vi "EventInPause_SM.vi"(0 "SM Private Data":refnum<class "Inspection Statemachine.lvclass">, 1 "LocalData_SM in":T1, 5 "Event Registration Refnum":refnum<event-registration>, 7 "CurrentState":string, 9 "Output Cluster":T2={"RackID"=0, "Trigger Light Camera Sequence"={"Light Sequence Trigger"="", "Status"="", "Mode"=""}, "Result Cluster"={"RackID"=0, "MeasurementValuesArray "=[], "ImagesArray"=[], "ResultPF"=FALSE, "ProductionCountDetails"={"TotalFail"=0, "TotalPass"=0, "TotalCount"=0}, "ReelCountDetails"={"ReelFail"=0, "ReelPass"=0, "ReelCount"=0}, "ControlPFArray"=[], "SpecificationPFArray"=[], "SpecificationFail"=FALSE, "ReelNumber"=0, "Status"=""}, "Analytics VI refnum"=refnum, "Statistical parameters "=[], "Sensor Name"="", "Camera Name"="", "PopupInput"={"Pop-up Type"=enum."Open Logo Display", "Title"="", "Message"="", "Button 1 Text"="", "Button 2 Text"="", "Show Close? T/F"=FALSE, "Title Blink? T/F"=FALSE, "Title Blink Colour"=0}, "PartInfo"={"PartName"="", "NumberOfRacks"=0, "TotalCount"=0, "ReelCount"=0, "OperatorName"="", "StampingMachineID"=0, "RackID"=0, "Reinitialize"=FALSE, "MeasurementNamesArray"=[], "MeasurementIDArray"=[], "SpecValuesArray"=[], "CameraNamesArray"=[]}, "StateMsgToMI"="", "InspectionStatusToMI"="", "StateMsgToRC"="", "StateMsgToUI"="", "StateMsgToDL"="", "StateMsgToAN"="", "StateMsgToSM"="", "EventData"={"EventName"="", "EventReason"=""}, "CameraOpticsDiagnosticsResult"={"LightCameraName"="", "DiagnosedImage"=refnum, "DustPercentage"=0.0, "Result"=TRUE}, "AllPartInfo"=[{"PartName"="", "NumberOfRacks"=0, "MeasurementIDsArray"=[], "MeasurementNamesArray"=[], "SpecValuesArray"=[]}], "SystemParameters"={"SystemName"="", "SystemID"="", "CustomerDetails"={"CustomerName"="", "CustomerId"="", "Location"="", "NumberOfShifts"=0.0, "ShiftDetails"=[]}, "InstallationDate"="", "NextServiceDate"="", "NumberOfRacks"=0, "TotalNumberOfCameras"=0, "SoftwareFeatures"={"HardwareEmulated"=FALSE, "PowerOnSelfTest"=FALSE, "DiagnosticsEnable"=FALSE, "AnalyticsEnable"=FALSE, "DefectTrackingEnable"=FALSE, "AutomaticGuideMovement"=FALSE, "DoorPokayokeEnable"=FALSE, "FailCountDisplayEnable"=FALSE, "FailCountReversalEnable"=FALSE, "DataLoggingEnable"=FALSE, "PauseOnReelCountFinish"=FALSE, "StopOnTotalCountFinish"=FALSE, "IoTEnable"=FALSE, "ReportEnable"=FALSE, "DebugLevel"=0.0, "PowerOnSelfTestFeatures"={"TimingUnit"=FALSE, "MachinePowerStatusCheck"=FALSE, "GuideMotor"=FALSE, "CameraOptics"=FALSE, "MasterSample"=FALSE}, "DiagnosticsFeatures"={"TimingUnit"=FALSE, "GuideMotor"=FALSE, "CameraOptics"=FALSE, "ReelerMotor"=FALSE, "HardwareButtons"=FALSE, "Sensors"=FALSE, "TowerLamp"=FALSE, "MasterSample"=FALSE}, "UserInterface"={"DynamicImageHandlingEnable"=FALSE, "DoorPokaYokeButtonVisible"=FALSE, "FailCountDisplayButtonVisible"=FALSE, "FailCountReversalButtonVisible"=FALSE}, "PopupOptions"={"ReasonForPause"=FALSE, "ReasonForFail"=FALSE, "ReasonForStop"=FALSE, "CpCpkOnReelFinish"=FALSE}, "DataloggingFeatures"={"EventData"=FALSE, "MeasurementData"=FALSE, "StatisticalData"=FALSE, "ReelData"=FALSE, "FailedMeasurementData"=FALSE, "FailedImages"=FALSE}, "IoT"={"SMSAlertEnable"=FALSE, "EmailAlertEnable"=FALSE}}}, "PartsConfigured"=[], "CameraSequenceList"=[], "SensorList"=[], "MasterSampleMessages"={"MasterSampleMessage"="", "PartMessage"=""}, "SensorDiagnosticsResult"={"Image Array"=[], "ImageCount"=0}, "IgnoredCountDetails"={"ReelCount"=0, "TotalCount"=0}, "MachineStatusToDL"="", "MasterSamplePartName"=""}, 11 "error in (no error)":errorcluster) -> (3 "LocalData_SM out":T1, 4 "NextState":string, 15 "error out":errorcluster)   [LabVIEW 2019, in "Inspection Statemachine.lvclass"]
uses:
  Inspection Statemachine.lvclass
  <vilib>/vision/Image Controls.llb/IMAQ Image.ctl
  Controls/Result Cluster_SM.ctl
  Common/Controls/Camera Optics Diagnostics Result.ctl
  Common/Controls/Pop-up Input.ctl
  Controls/Output Cluster_SM.ctl
  Common/Controls/AllPartInfo.ctl
  Controls/LocalData_SM.ctl
  Common/Controls/Diagnostics Result.ctl
  <vilib>/ActorFramework/Message Enqueuer/Message Enqueuer.lvclass
  Common/Controls/Acknowledgement.ctl
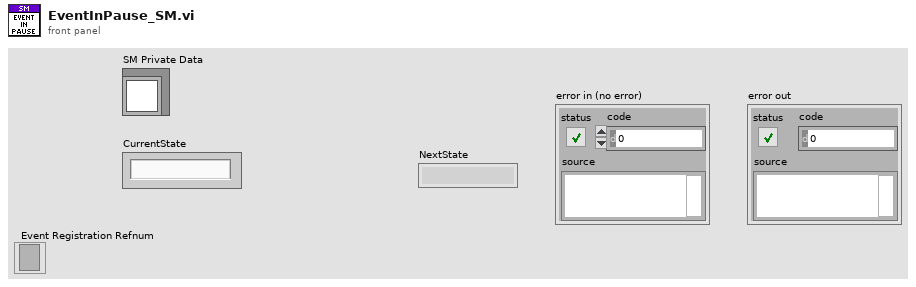
[diagram p1: front panel]
types:
  T1 = typedef "Inspection Statemachine.lvclass/LocalData_SM.ctl" = cluster{"Timeout":i32, "Core":cluster{"Current VI Reference":refnum<vi>, "Close Panel on Exit?":bool}, "Ack":u8, " CurrentState":string, "DirectExit":bool, "SoftwareExit":bool, "SensorDiagnosticsStatus":bool, "OutputCluster":T2, "SelComplete":bool, "ResultToMI":bool, "Exit":bool, "NumberOfActorsLaunched":i32, "BatchStart":bool, "LoadingBarActive":bool, "UpdateInPause":bool, " EventReason":string, "PopUpCategory":string, "PopUpActive":bool, "MasterSampleState":string, "CameraOpticsDiagnosticsStatus":bool, "CameraIndex":i32, "SensorIndex":i32}
  T2 = typedef "Inspection Statemachine.lvclass/Output Cluster_SM.ctl" = cluster{"RackID":u8, "Trigger Light Camera Sequence":cluster{"Light Sequence Trigger":string, "Status":string, "Mode":string}, "Result Cluster":T3, "Analytics VI refnum":refnum<vi>, "Statistical parameters ":string[][], "Sensor Name":string, "Camera Name":string, "PopupInput":T5, "PartInfo":cluster{"PartName":string, "NumberOfRacks":u8, "TotalCount":u64, "ReelCount":u64, "OperatorName":string, "StampingMachineID":u32, "RackID":u8, "Reinitialize":bool, "MeasurementNamesArray":string[], "MeasurementIDArray":u16[], "SpecValuesArray":cluster{"LCL":dbl, "UCL":dbl, "LSL":dbl, "USL":dbl, "Nominal Value":dbl}[], "CameraNamesArray":string[]}, "StateMsgToMI":string, "InspectionStatusToMI":string, "StateMsgToRC":string, "StateMsgToUI":string, "StateMsgToDL":string, "StateMsgToAN":string, "StateMsgToSM":string, "EventData":cluster{"EventName":string, "EventReason":string}, "CameraOpticsDiagnosticsResult":T6, "AllPartInfo":T7, "SystemParameters":cluster{"SystemName":string, "SystemID":string, "CustomerDetails":cluster{"CustomerName":string, "CustomerId":string, "Location":string, "NumberOfShifts":dbl, "ShiftDetails":cluster{"Name":string, "Timing":string}[]}, "InstallationDate":string, "NextServiceDate":string, "NumberOfRacks":u8, "TotalNumberOfCameras":u8, "SoftwareFeatures":cluster{"HardwareEmulated":bool, "PowerOnSelfTest":bool, "DiagnosticsEnable":bool, "AnalyticsEnable":bool, "DefectTrackingEnable":bool, "AutomaticGuideMovement":bool, "DoorPokayokeEnable":bool, "FailCountDisplayEnable":bool, "FailCountReversalEnable":bool, "DataLoggingEnable":bool, "PauseOnReelCountFinish":bool, "StopOnTotalCountFinish":bool, "IoTEnable":bool, "ReportEnable":bool, "DebugLevel":dbl, "PowerOnSelfTestFeatures":cluster{"TimingUnit":bool, "MachinePowerStatusCheck":bool, "GuideMotor":bool, "CameraOptics":bool, "MasterSample":bool}, "DiagnosticsFeatures":cluster{"TimingUnit":bool, "GuideMotor":bool, "CameraOptics":bool, "ReelerMotor":bool, "HardwareButtons":bool, "Sensors":bool, "TowerLamp":bool, "MasterSample":bool}, "UserInterface":cluster{"DynamicImageHandlingEnable":bool, "DoorPokaYokeButtonVisible":bool, "FailCountDisplayButtonVisible":bool, "FailCountReversalButtonVisible":bool}, "PopupOptions":cluster{"ReasonForPause":bool, "ReasonForFail":bool, "ReasonForStop":bool, "CpCpkOnReelFinish":bool}, "DataloggingFeatures":cluster{"EventData":bool, "MeasurementData":bool, "StatisticalData":bool, "ReelData":bool, "FailedMeasurementData":bool, "FailedImages":bool}, "IoT":cluster{"SMSAlertEnable":bool, "EmailAlertEnable":bool}}}, "PartsConfigured":cluster{"Name":string, "NumberOfRack":u8}[], "CameraSequenceList":cluster{"Name":string, "RackID":u8}[], "SensorList":cluster{"Name":string, "RackID":u8}[], "MasterSampleMessages":cluster{"MasterSampleMessage":string, "PartMessage":string}, "SensorDiagnosticsResult":cluster{"Image Array":T4[], "ImageCount":u64}, "IgnoredCountDetails":cluster{"ReelCount":u64, "TotalCount":u64}, "MachineStatusToDL":string, "MasterSamplePartName":string}
  T3 = typedef "Inspection Statemachine.lvclass/Result Cluster_SM.ctl" = cluster{"RackID":u8, "MeasurementValuesArray ":dbl[], "ImagesArray":T4[], "ResultPF":bool, "ProductionCountDetails":cluster{"TotalFail":u64, "TotalPass":u64, "TotalCount":u64}, "ReelCountDetails":cluster{"ReelFail":u64, "ReelPass":u64, "ReelCount":u64}, "ControlPFArray":bool[], "SpecificationPFArray":bool[], "SpecificationFail":bool, "ReelNumber":u64, "Status":string}
  T4 = typedef "IMAQ Image.ctl" = refnum<image>
  T5 = typedef "Pop-up Input.ctl" = cluster{"Pop-up Type":enum16{"Open Logo Display", "Close Logo Display", "Open Loading Bar", "Close Loading Bar", "Open Alert Display", "Close Alert Display", "One button dialog box", "Two button dialog box", "User Authentication"}, "Title":string, "Message":string, "Button 1 Text":string, "Button 2 Text":string, "Show Close? T/F":bool, "Title Blink? T/F":bool, "Title Blink Colour":u32}
  T6 = typedef "Camera Optics Diagnostics Result.ctl" = cluster{"LightCameraName":string, "DiagnosedImage":T4, "DustPercentage":dbl, "Result":bool}
  T7 = typedef "AllPartInfo.ctl" = cluster{"PartName":string, "NumberOfRacks":u8, "MeasurementIDsArray":u16[], "MeasurementNamesArray":string[], "SpecValuesArray":cluster{"LCL":dbl, "UCL":dbl, "LSL":dbl, "USL":dbl, "NominalValue":dbl}[]}[]
  T8 = enum16{"Open Logo Display", "Close Logo Display", "Open Loading Bar", "Close Loading Bar", "Open Alert Display", "Close Alert Display", "One button dialog box", "Two button dialog box", "User Authentication"}
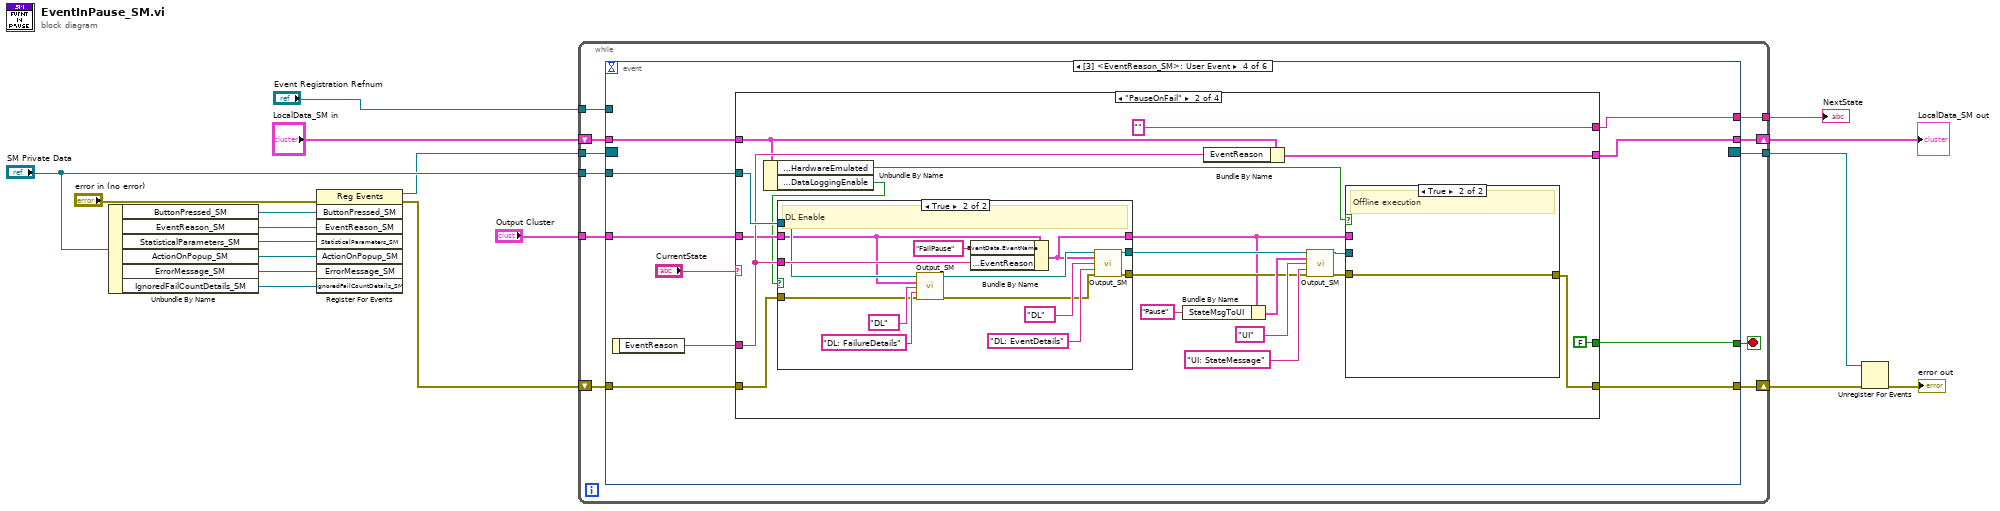
[diagram p0: block diagram]
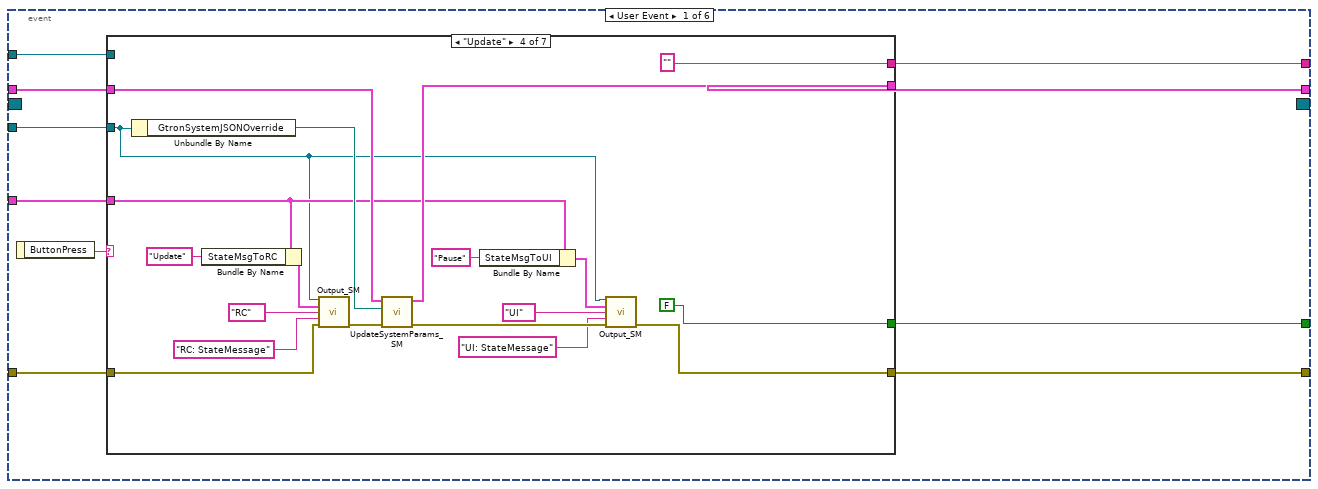
[diagram p2: hidden frame]
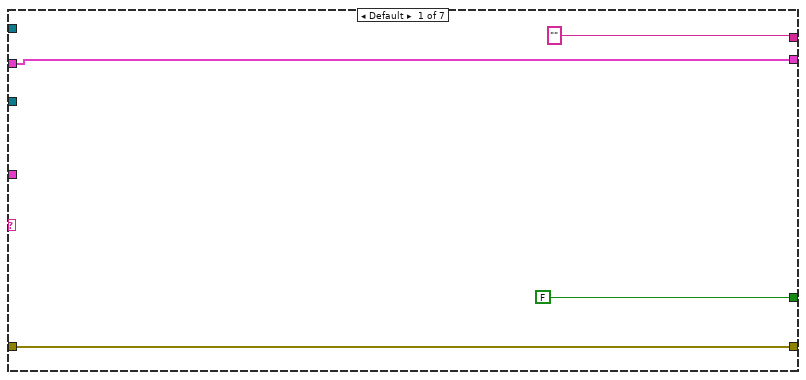
[diagram p3: hidden frame]
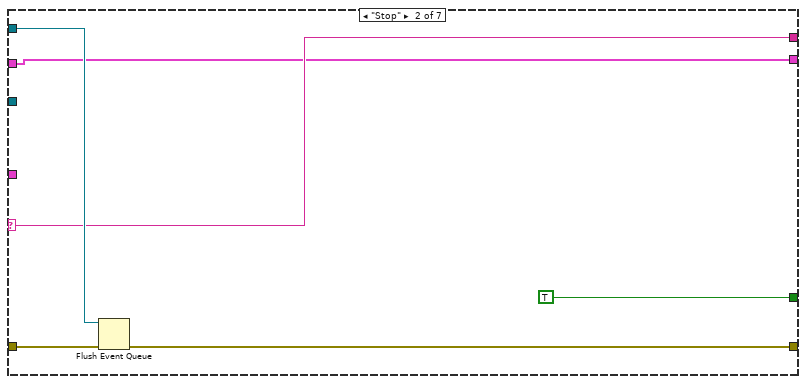
[diagram p4: hidden frame]
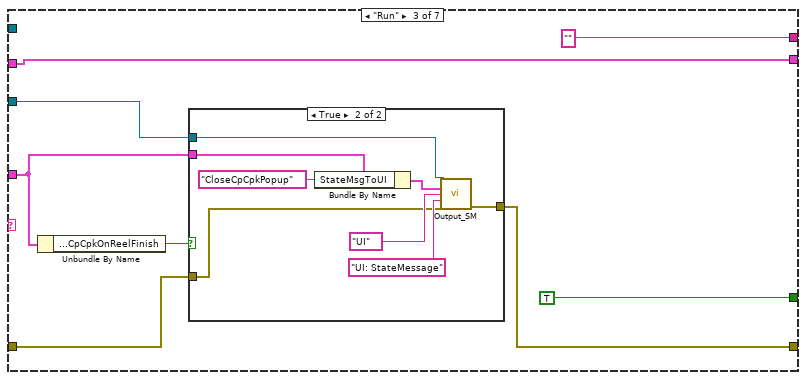
[diagram p5: hidden frame]
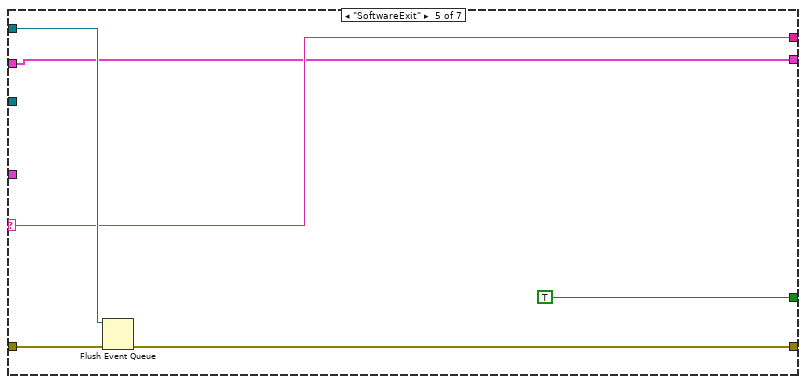
[diagram p7: hidden frame]
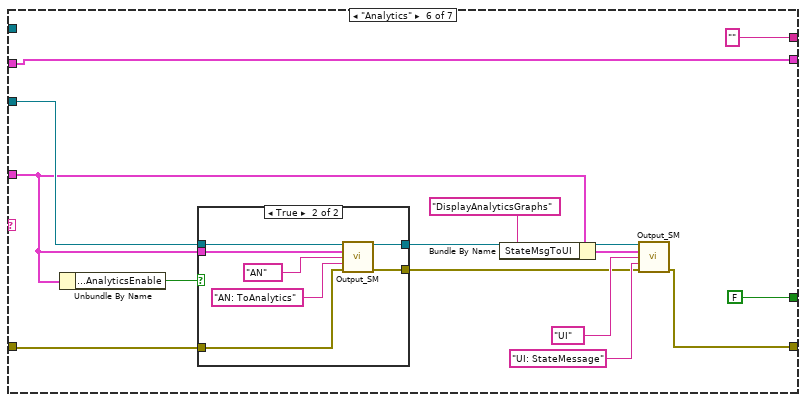
[diagram p8: hidden frame]
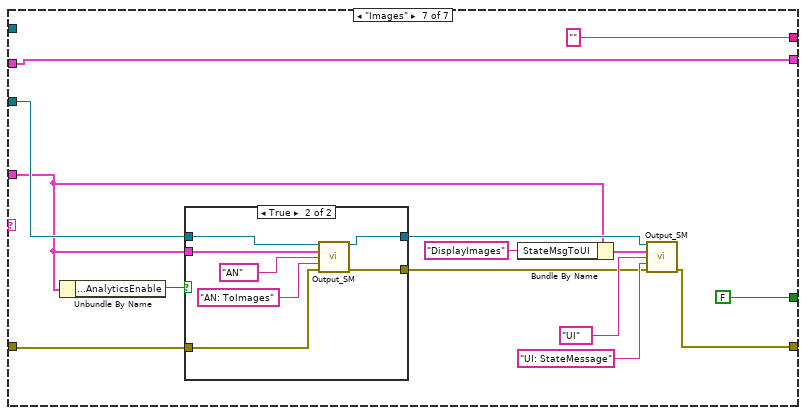
[diagram p10: hidden frame]
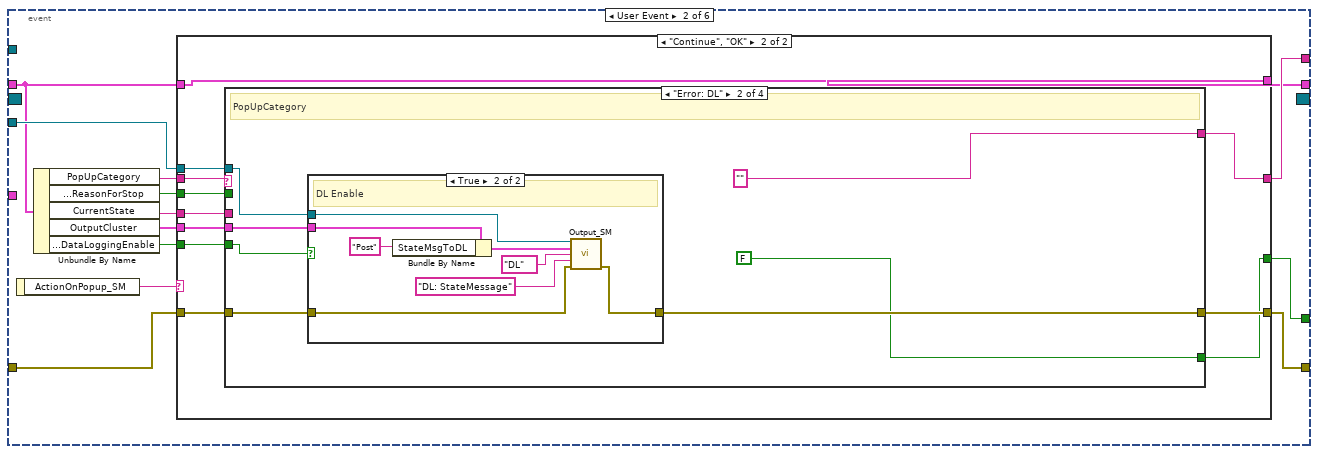
[diagram p12: hidden frame]
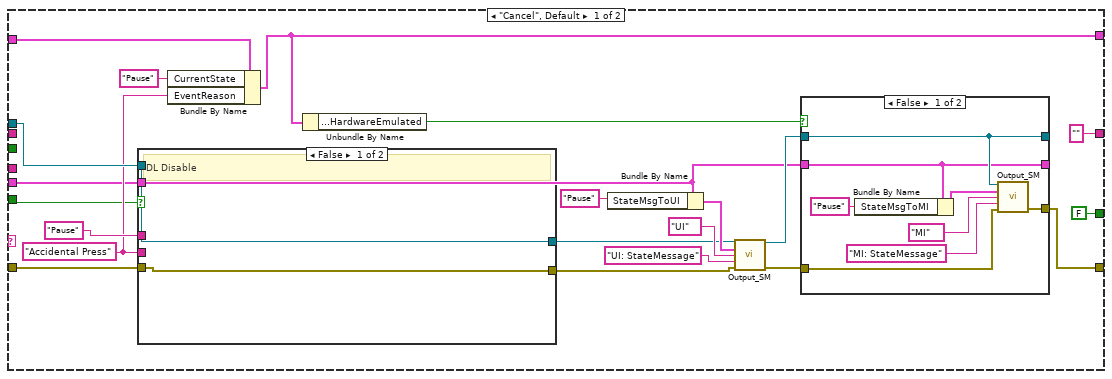
[diagram p13: hidden frame]
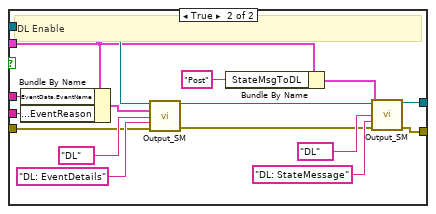
[diagram p14: hidden frame]
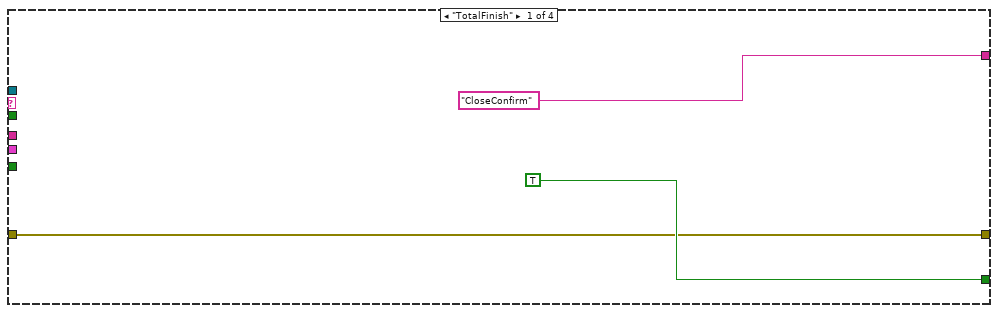
[diagram p16: hidden frame]
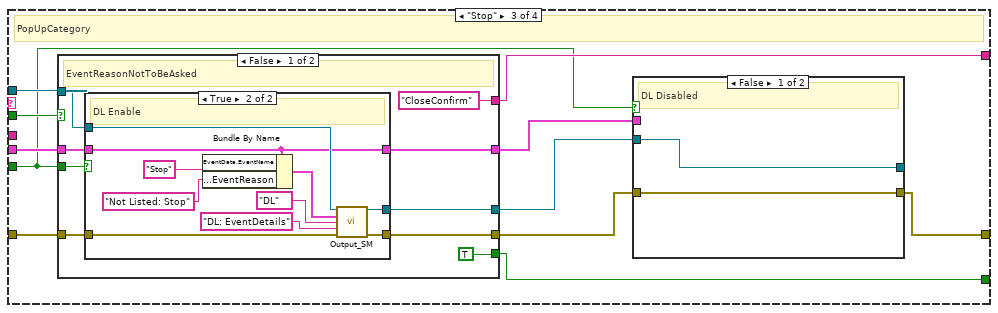
[diagram p18: hidden frame]
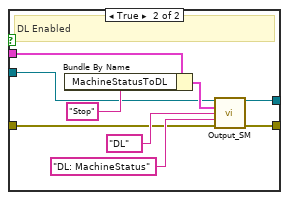
[diagram p19: hidden frame]
diagram:
  n1 = Unbundle By Name("SM Private Data") -> ("ButtonPressed_SM"=w14:refnum<user-event>, "EventReason_SM"=w13:refnum<user-event>, "StatisticalParameters_SM"=w12:refnum<user-event>, "ActionOnPopup_SM"=w4:refnum<user-event>, "ErrorMessage_SM"=w2:refnum<user-event>, "IgnoredFailCountDetails_SM"=w1:refnum<user-event>)
  n2 = register-events(error in="error in (no error)", w14, w13, w12, w4, w2, w1) -> (reference out=w10:refnum<event-registration>, error out=w8:errorcluster)  [unwired: 1 in]
  n3 = while {
    tunnel: w10 -> [w29]
    tunnel: [w28] -> w17
    tunnel: [w23] -> w18
    tunnel: "Event Registration Refnum" -> [w24]
    tunnel: "SM Private Data" -> [w22]
    tunnel: "Output Cluster" -> [w21]
    shift-right: [w25] -> w16
    shift-left: w8 -> [w26]
    shift-right: [w19] -> w5
    shift-left: "LocalData_SM in" -> [w20]
    stop <- w27 stop-if-true
    n4 = event shown="[3] <EventReason_SM>: User Event" {
      selector: w29 -> [_ _ _ _ _ _]
      dyn-events: [_ _ _ _ _ _] -> w28
      timeout: _ -> [_ _ _ _ _ _]
      tunnel: [w35 w142 FALSE w323 _ FALSE] -> w27
      tunnel: w26 -> [w39 w149 w298 w327 w439 w488]
      tunnel: [w38 w150 w297 w324 w443 w487] -> w25
      tunnel: w24 -> [w36 _ _ _ _ _]
      tunnel: [w34 w143 "" w322 "" ""] -> w23
      tunnel: w22 -> [w33 w144 w296 w326 w440 w485]
      tunnel: w21 -> [w32 _ w299 w325 w448 _]
      tunnel: w20 -> [w31 w141 w292 w321 w452 w484]
      tunnel: [w30 w140 w291 w320 w452 w484] -> w19
      event User Event {
        n5 = event-data() -> ("ButtonPress"=w37:string)  [unwired: 1 in]
        n6 = case shown="\"Update\"" w37 {
          selector: w37 -> [_ w46 _ _ w87 _ _]
          tunnel: w39 -> [w43 w49 w52 w84 w90 w101 w124]
          tunnel: [w43 w45 w51 w73 w89 w100 w123] -> w38
          tunnel: w36 -> [_ w48 _ _ w88 _ _]
          tunnel: [FALSE TRUE TRUE FALSE TRUE FALSE FALSE] -> w35
          tunnel: ["" w46 "" "" w87 "" ""] -> w34
          tunnel: w33 -> [_ _ w53 w67 _ w95 w118]
          tunnel: w32 -> [_ _ w50 w71 _ w93 w116]
          tunnel: w31 -> [w40 w44 w55 w77 w86 w96 w119]
          tunnel: [w40 w44 w55 w76 w86 w96 w119] -> w30
          frame Default {
          }
          frame "Stop" {
            n7 = Flush Event Queue(0:w48, 3:w49) -> (11:w45:errorcluster)  [unwired: 4 in, 2 out]
          }
          frame "Run" {
            n8 = Unbundle By Name(w50) -> ("SystemParameters.SoftwareFeatures.PopupOptions.CpCpkOnReelFinish"=w54:bool)
            n9 = case shown="True" w54 {
              tunnel: w53 -> [_ w64]
              tunnel: w52 -> [w58 w63]
              tunnel: [w58 w62] -> w51
              tunnel: w50 -> [_ w61]
              frame False {
              }
              frame True {
                n10 = Bundle By Name(cluster=w61, "StateMsgToUI"="CloseCpCpkPopup" ("StateMsgToSM")) -> (w60:T2)
                n11 = call "Output_SM.vi"("SM Private Data in"=w64, "Output Cluster"=w60, "Receiver Name"="UI", "State"="UI: StateMessage", "error in (no error)"=w63) -> ("error out"=w62:errorcluster)  [unwired: 9 in, 1 out]
              }
            }
          }
          frame "Update" {
            n12 = Unbundle By Name(w67) -> ("GtronSystemJSONOverride"=w75:path)
            n13 = Bundle By Name(cluster=w71, "StateMsgToRC"="Update") -> (w81:T2)
            n14 = call "Output_SM.vi"("SM Private Data in"=w67, "Output Cluster"=w81, "Receiver Name"="RC", "State"="RC: StateMessage", "error in (no error)"=w84) -> ("error out"=w78:errorcluster)  [unwired: 9 in, 1 out]
            n15 = call "UpdateSystemParams_SM.vi"("error in (no error)"=w78, "Override File Path"=w75, "Cluster In"=w77) -> ("error out"=w74:errorcluster, "Cluster Out"=w76:T1)  [unwired: 7 in]
            n16 = Bundle By Name(cluster=w71, "StateMsgToUI"="Pause") -> (w70:T2)
            n17 = call "Output_SM.vi"("SM Private Data in"=w67, "Output Cluster"=w70, "Receiver Name"="UI", "State"="UI: StateMessage", "error in (no error)"=w74) -> ("error out"=w73:errorcluster)  [unwired: 9 in, 1 out]
          }
          frame "SoftwareExit" {
            n18 = Flush Event Queue(0:w88, 3:w90) -> (11:w89:errorcluster)  [unwired: 4 in, 2 out]
          }
          frame "Analytics" {
            n19 = Unbundle By Name(w93) -> ("SystemParameters.SoftwareFeatures.AnalyticsEnable"=w92:bool)
            n20 = case shown="True" w92 {
              tunnel: [w106 w114] -> w103
              tunnel: w101 -> [w106 w111]
              tunnel: w95 -> [w107 w110]
              tunnel: w93 -> [_ w109]
              tunnel: [w107 w108] -> w94
              frame False {
              }
              frame True {
                n21 = call "Output_SM.vi"("SM Private Data in"=w110, "Output Cluster"=w109, "Receiver Name"="AN", "State"="AN: ToAnalytics", "error in (no error)"=w111) -> ("SM Private Data out"=w108:refnum<class "Inspection Statemachine.lvclass">, "error out"=w114:errorcluster)  [unwired: 9 in]
              }
            }
            n22 = Bundle By Name(cluster=w93, "StateMsgToUI"="DisplayAnalyticsGraphs") -> (w97:T2)
            n23 = call "Output_SM.vi"("SM Private Data in"=w94, "Output Cluster"=w97, "Receiver Name"="UI", "State"="UI: StateMessage", "error in (no error)"=w103) -> ("error out"=w100:errorcluster)  [unwired: 9 in, 1 out]
          }
          frame "Images" {
            n24 = Unbundle By Name(w116) -> ("SystemParameters.SoftwareFeatures.AnalyticsEnable"=w115:bool)
            n25 = case shown="True" w115 {
              tunnel: [w129 w137] -> w126
              tunnel: w124 -> [w129 w134]
              tunnel: w116 -> [_ w133]
              tunnel: w118 -> [w130 w132]
              tunnel: [w130 w131] -> w117
              frame False {
              }
              frame True {
                n26 = call "Output_SM.vi"("SM Private Data in"=w132, "Output Cluster"=w133, "Receiver Name"="AN", "State"="AN: ToImages", "error in (no error)"=w134) -> ("SM Private Data out"=w131:refnum<class "Inspection Statemachine.lvclass">, "error out"=w137:errorcluster)  [unwired: 9 in]
              }
            }
            n27 = Bundle By Name(cluster=w116, "StateMsgToUI"="DisplayImages") -> (w120:T2)
            n28 = call "Output_SM.vi"("SM Private Data in"=w117, "Output Cluster"=w120, "Receiver Name"="UI", "State"="UI: StateMessage", "error in (no error)"=w126) -> ("error out"=w123:errorcluster)  [unwired: 9 in, 1 out]
          }
        }
      }
      event User Event {
        n29 = event-data() -> ("ActionOnPopup_SM"=w148:string)  [unwired: 1 in]
        n30 = Unbundle By Name(w141) -> ("PopUpCategory"=w139:string, "OutputCluster.SystemParameters.SoftwareFeatures.PopupOptions.ReasonForStop"=w145:bool, "CurrentState"=w146:string, "OutputCluster"=w147:T2, "OutputCluster.SystemParameters.SoftwareFeatures.DataLoggingEnable"=w138:bool)
        n31 = case shown="\"Continue\", \"OK\"" w148 {
          tunnel: ["" w211] -> w143
          tunnel: w146 -> [_ w210]
          tunnel: w147 -> [w153 w209]
          tunnel: w144 -> [w161 w208]
          tunnel: w149 -> [w162 w207]
          tunnel: [w155 w206] -> w150
          tunnel: w145 -> [_ w205]
          tunnel: [FALSE w204] -> w142
          tunnel: w141 -> [w165 w203]
          tunnel: [w157 w203] -> w140
          tunnel: w139 -> [_ w202]
          tunnel: w138 -> [w151 w201]
          frame "Cancel", Default {
            w160 = "Accidental Press" ("EventReason")
            n32 = case shown="False" w151 {
              tunnel: "Pause" ("DataLogger.EventDetails.EventName") -> [_ w187]
              tunnel: w162 -> [w172 w185]
              tunnel: w161 -> [w173 w184]
              tunnel: w160 -> [_ w183]
              tunnel: [w173 w177] -> w154
              tunnel: w153 -> [_ w175]
              tunnel: [w172 w174] -> w152
              frame False {
                # "DL Disable"
              }
              frame True {
                # "DL Enable"
                n33 = Bundle By Name(cluster=w175, "EventData.EventName"=w187, "EventData.EventReason"=w183) -> (w188:T2)
                n34 = call "Output_SM.vi"("SM Private Data in"=w184, "Output Cluster"=w188, "Receiver Name"="DL", "State"="DL: EventDetails", "error in (no error)"=w185) -> ("SM Private Data out"=w178:refnum<class "Inspection Statemachine.lvclass">, "error out"=w176:errorcluster)  [unwired: 9 in]
                n35 = Bundle By Name(cluster=w175, "StateMsgToDL"="Post") -> (w180:T2)
                n36 = call "Output_SM.vi"("SM Private Data in"=w178, "Output Cluster"=w180, "Receiver Name"="DL", "State"="DL: StateMessage", "error in (no error)"=w176) -> ("SM Private Data out"=w177:refnum<class "Inspection Statemachine.lvclass">, "error out"=w174:errorcluster)  [unwired: 9 in]
              }
            }
            n37 = Bundle By Name(cluster=w165, "CurrentState"="Pause", "EventReason"=w160) -> (w157:T1)
            n38 = Unbundle By Name(w157) -> ("OutputCluster.SystemParameters.SoftwareFeatures.HardwareEmulated"=w156:bool)
            n39 = Bundle By Name(cluster=w153, "StateMsgToUI"="Pause" ("StateMsgToRC")) -> (w167:T2)
            n40 = call "Output_SM.vi"("SM Private Data in"=w154, "Output Cluster"=w167, "Receiver Name"="UI", "State"="UI: StateMessage", "error in (no error)"=w152) -> ("SM Private Data out"=w158:refnum<class "Inspection Statemachine.lvclass">, "error out"=w159:errorcluster)  [unwired: 9 in]
            n41 = case shown="False" w156 {
              tunnel: w153 -> [w190 w198]
              tunnel: w158 -> [w191 w199]
              tunnel: w159 -> [w193 w200]
              tunnel: [w192 w200] -> w155
              tunnel: [w191 w199] -> _
              tunnel: [w190 w198] -> _
              frame False {
                n42 = Bundle By Name(cluster=w190, "StateMsgToMI"="Pause") -> (w195:T2)
                n43 = call "Output_SM.vi"("SM Private Data in"=w191, "Output Cluster"=w195, "Receiver Name"="MI", "State"="MI: StateMessage", "error in (no error)"=w193) -> ("error out"=w192:errorcluster)  [unwired: 9 in, 1 out]
              }
              frame True {
              }
            }
          }
          frame "Continue", "OK" {
            n44 = case shown="\"Error: DL\"" w202 {
              tunnel: ["CloseConfirm" "" w241 ""] -> w211
              tunnel: w210 -> [_ _ _ _]
              tunnel: w209 -> [_ w220 w240 _]
              tunnel: w208 -> [_ w219 w239 _]
              tunnel: w207 -> [w212 w218 w238 w288]
              tunnel: [w212 w217 w235 w288] -> w206
              tunnel: w205 -> [_ _ w237 _]
              tunnel: [TRUE FALSE w236 FALSE] -> w204
              tunnel: w201 -> [_ w215 w231 _]
              frame "TotalFinish" {
              }
              frame "Error: DL" {
                # "PopUpCategory"
                n45 = case shown="True" w215 {
                  tunnel: w220 -> [_ w230]
                  tunnel: w219 -> [_ w229]
                  tunnel: w218 -> [w222 w228]
                  tunnel: [w222 w227] -> w217
                  frame False {
                    # "DL DIsable"
                  }
                  frame True {
                    # "DL Enable"
                    n46 = Bundle By Name(cluster=w230, "StateMsgToDL"="Post") -> (w225:T2)
                    n47 = call "Output_SM.vi"("SM Private Data in"=w229, "Output Cluster"=w225, "Receiver Name"="DL", "State"="DL: StateMessage", "error in (no error)"=w228) -> ("error out"=w227:errorcluster)  [unwired: 9 in, 1 out]
                  }
                }
              }
              frame "Stop" {
                # "PopUpCategory"
                n48 = case shown="False" w237 {
                  tunnel: w238 -> [w259 w277]
                  tunnel: [w260 w284] -> w234
                  tunnel: w240 -> [w258 w275]
                  tunnel: w239 -> [w261 w278]
                  tunnel: ["CloseConfirm" ""] -> w241
                  tunnel: [TRUE FALSE] -> w236
                  tunnel: w231 -> [w255 _]
                  tunnel: [w254 w276] -> w233
                  tunnel: [w253 w275] -> w232
                  frame False {
                    # "EventReasonNotToBeAsked"
                    n49 = case shown="True" w255 {
                      tunnel: w261 -> [w262 w270]
                      tunnel: [w264 w269] -> w260
                      tunnel: w259 -> [w264 w268]
                      tunnel: w258 -> [w263 w265]
                      tunnel: [w262 w266] -> w254
                      tunnel: [w263 w265] -> w253
                      frame False {
                        # "DL Disable"
                      }
                      frame True {
                        # "DL Enable"
                        n50 = Bundle By Name(cluster=w265, "EventData.EventName"="Stop" ("DataLogger.EventDetails.EventName"), "EventData.EventReason"="Not Listed: Stop") -> (w272:T2)
                        n51 = call "Output_SM.vi"("SM Private Data in"=w270, "Output Cluster"=w272, "Receiver Name"="DL", "State"="DL: EventDetails", "error in (no error)"=w268) -> ("SM Private Data out"=w266:refnum<class "Inspection Statemachine.lvclass">, "error out"=w269:errorcluster)  [unwired: 9 in]
                      }
                    }
                  }
                  frame True {
                    # "EventReasonToBeAsked"
                    n52 = Bundle By Name(cluster=w275, "StateMsgToUI"="Stop") -> (w282:T2)
                    n53 = call "Output_SM.vi"("SM Private Data in"=w278, "Output Cluster"=w282, "Receiver Name"="UI", "State"="UI: AskEventReason", "error in (no error)"=w277) -> ("SM Private Data out"=w276:refnum<class "Inspection Statemachine.lvclass">, "error out"=w284:errorcluster)  [unwired: 9 in]
                  }
                }
                n54 = case shown="False" w231 {
                  tunnel: w234 -> [w242 w248]
                  tunnel: w233 -> [w243 w247]
                  tunnel: w232 -> [_ w246]
                  tunnel: [w242 w245] -> w235
                  tunnel: [w243 w244] -> _
                  frame False {
                    # "DL Disabled"
                  }
                  frame True {
                    # "DL Enabled"
                    n55 = Bundle By Name(cluster=w246, "MachineStatusToDL"="Stop" ("StateMsgToDL")) -> (w251:T2)
                    n56 = call "Output_SM.vi"("SM Private Data in"=w247, "Output Cluster"=w251, "Receiver Name"="DL", "State"="DL: MachineStatus", "error in (no error)"=w248) -> ("SM Private Data out"=w244:refnum<class "Inspection Statemachine.lvclass">, "error out"=w245:errorcluster)  [unwired: 9 in]
                  }
                }
              }
              frame Default {
              }
            }
          }
        }
      }
      event User Event {
        n57 = event-data() -> ("ErrorMessage"=w294:string)  [unwired: 1 in]
        n58 = Match Pattern(string=w294, regular expression="_") -> (before substring=w293:string)  [unwired: 1 in, 3 out]
        n59 = case shown="\"DataLogger\"" w293 {
          tunnel: w299 -> [_ w304]
          tunnel: w298 -> [w300 w311]
          tunnel: [w300 w310] -> w297
          tunnel: w296 -> [_ w309]
          tunnel: w292 -> [w301 w306]
          tunnel: [w301 w305] -> w291
          frame Default {
          }
          frame "DataLogger" {
            n60 = Bundle By Name(cluster=w306, "DirectExit"=FALSE ("Direct Exit"), "SoftwareExit"=FALSE ("Software Exit?"), "PopUpCategory"="Error: DL", "PopUpActive"=TRUE) -> (w305:T1)
            n61 = Bundle By Name(cluster=w304, "PopupInput.Title"="ALERT!" ("title"), "PopupInput.Message"="File Open!\nUnable To Write.Please Close Data File." ("string"), "PopupInput.Title Blink? T/F"=TRUE ("title blink?"), "PopupInput.Button 1 Text"="OK", "PopupInput.Pop-up Type"=T8."One button dialog box") -> (w314:T2)
            n62 = call "Output_SM.vi"("SM Private Data in"=w309, "Output Cluster"=w314, "Receiver Name"="UI", "State"="UI: DisplayPopup", "error in (no error)"=w311) -> ("error out"=w310:errorcluster)  [unwired: 9 in, 1 out]
          }
        }
      }
      event User Event {
        n63 = event-data() -> ("EventReason"=w328:string)  [unwired: 1 in]
        n64 = case shown="\"PauseOnFail\"" "CurrentState" {
          tunnel: w328 -> [w333 w359 w402 _]
          tunnel: w327 -> [w334 w368 w413 w438]
          tunnel: w326 -> [w335 w367 w412 _]
          tunnel: w325 -> [w331 w352 w397 _]
          tunnel: [w338 w354 w400 w438] -> w324
          tunnel: [TRUE FALSE FALSE FALSE] -> w323
          tunnel: ["CloseConfirm" "" "" ""] -> w322
          tunnel: w321 -> [w332 w358 w403 w435]
          tunnel: [w332 w360 w399 w435] -> w320
          frame "Stop" {
            n65 = Unbundle By Name(w331) -> ("SystemParameters.SoftwareFeatures.DataLoggingEnable"=w330:bool)
            n66 = case shown="False" w330 {
              tunnel: [w339 w344] -> w338
              tunnel: w335 -> [_ w343]
              tunnel: w331 -> [_ w342]
              tunnel: w334 -> [w339 w341]
              tunnel: w333 -> [_ w340]
              frame False {
                # "DL Disable"
              }
              frame True {
                # "DL Enable"
                n67 = Bundle By Name(cluster=w342, "EventData.EventName"="Stop" ("DataLogger.EventDetails.EventName"), "EventData.EventReason"=w340) -> (w346:T2)
                n68 = call "Output_SM.vi"("SM Private Data in"=w343, "Output Cluster"=w346, "Receiver Name"="DL", "State"="DL: EventDetails", "error in (no error)"=w341) -> ("error out"=w344:errorcluster)  [unwired: 9 in, 1 out]
              }
            }
          }
          frame "PauseOnFail" {
            n69 = Unbundle By Name(w358) -> ("OutputCluster.SystemParameters.SoftwareFeatures.HardwareEmulated"=w357:bool, "OutputCluster.SystemParameters.SoftwareFeatures.DataLoggingEnable"=w350:bool)
            n70 = case shown="True" w350 {
              tunnel: w368 -> [w371 w377]
              tunnel: w367 -> [w369 w375]
              tunnel: w359 -> [_ w382]
              tunnel: [w369 w380] -> w353
              tunnel: w352 -> [w370 w373]
              tunnel: [w371 w381] -> w351
              tunnel: [w370 w372] -> w349
              frame False {
                # "DL Disable"
              }
              frame True {
                # "DL Enable"
                n71 = call "Output_SM.vi"("SM Private Data in"=w375, "Output Cluster"=w373, "Receiver Name"="DL", "State"="DL: FailureDetails", "error in (no error)"=w377) -> ("SM Private Data out"=w374:refnum<class "Inspection Statemachine.lvclass">, "error out"=w376:errorcluster)  [unwired: 9 in]
                n72 = Bundle By Name(cluster=w373, "EventData.EventName"="FailPause" ("DataLogger.EventDetails.EventName"), "EventData.EventReason"=w382) -> (w372:T2)
                n73 = call "Output_SM.vi"("SM Private Data in"=w374, "Output Cluster"=w372, "Receiver Name"="DL", "State"="DL: EventDetails", "error in (no error)"=w376) -> ("SM Private Data out"=w380:refnum<class "Inspection Statemachine.lvclass">, "error out"=w381:errorcluster)  [unwired: 9 in]
              }
            }
            n74 = Bundle By Name(cluster=w349, "StateMsgToUI"="Pause") -> (w365:T2)
            n75 = Bundle By Name(cluster=w358, "EventReason"=w359) -> (w360:T1)
            n76 = call "Output_SM.vi"("SM Private Data in"=w353, "Output Cluster"=w365, "Receiver Name"="UI", "State"="UI: StateMessage", "error in (no error)"=w351) -> ("SM Private Data out"=w356:refnum<class "Inspection Statemachine.lvclass">, "error out"=w355:errorcluster)  [unwired: 9 in]
            n77 = case shown="True" w357 {
              tunnel: w356 -> [w389 _]
              tunnel: w349 -> [w388 _]
              tunnel: w355 -> [w387 w394]
              tunnel: [w386 w394] -> w354
              frame False {
                # "Online execution"
                n78 = Bundle By Name(cluster=w388, "StateMsgToMI"="Pause") -> (w391:T2)
                n79 = call "Output_SM.vi"("SM Private Data in"=w389, "Output Cluster"=w391, "Receiver Name"="MI", "State"="MI: StateMessage", "error in (no error)"=w387) -> ("error out"=w386:errorcluster)  [unwired: 9 in, 1 out]
              }
              frame True {
                # "Offline execution"
              }
            }
          }
          frame "Pause" {
            n80 = Bundle By Name(cluster=w403, "EventReason"=w402) -> (w399:T1)
            n81 = Unbundle By Name(w399) -> ("OutputCluster.SystemParameters.SoftwareFeatures.HardwareEmulated"=w398:bool, "OutputCluster.SystemParameters.SoftwareFeatures.DataLoggingEnable"=w395:bool)
            n82 = case shown="True" w395 {
              tunnel: w413 -> [w414 w423]
              tunnel: w412 -> [w415 w421]
              tunnel: [w415 w419] -> w407
              tunnel: [w414 w418] -> w406
              tunnel: w402 -> [_ w417]
              tunnel: w397 -> [_ w416]
              frame False {
                # "DL Disable"
              }
              frame True {
                # "DL Enable"
                n83 = Bundle By Name(cluster=w416, "EventData.EventName"="Pause" ("DataLogger.EventDetails.EventName"), "EventData.EventReason"=w417) -> (w422:T2)
                n84 = call "Output_SM.vi"("SM Private Data in"=w421, "Output Cluster"=w422, "Receiver Name"="DL", "State"="DL: EventDetails", "error in (no error)"=w423) -> ("SM Private Data out"=w419:refnum<class "Inspection Statemachine.lvclass">, "error out"=w418:errorcluster)  [unwired: 9 in]
              }
            }
            n85 = Bundle By Name(cluster=w397, "StateMsgToUI"="Pause") -> (w410:T2)
            n86 = call "Output_SM.vi"("SM Private Data in"=w407, "Output Cluster"=w410, "Receiver Name"="UI", "State"="UI: StateMessage", "error in (no error)"=w406) -> ("SM Private Data out"=w396:refnum<class "Inspection Statemachine.lvclass">, "error out"=w401:errorcluster)  [unwired: 9 in]
            n87 = case shown="True" w398 {
              tunnel: w396 -> [w429 _]
              tunnel: w397 -> [w428 _]
              tunnel: w401 -> [w427 w434]
              tunnel: [w426 w434] -> w400
              frame False {
                # "Online execution"
                n88 = Bundle By Name(cluster=w428, "StateMsgToMI"="Pause") -> (w431:T2)
                n89 = call "Output_SM.vi"("SM Private Data in"=w429, "Output Cluster"=w431, "Receiver Name"="MI", "State"="MI: StateMessage", "error in (no error)"=w427) -> ("error out"=w426:errorcluster)  [unwired: 9 in, 1 out]
              }
              frame True {
                # "Offline execution"
              }
            }
          }
          frame Default {
          }
        }
      }
      event User Event {
        n90 = event-data() -> ("StatisticalParameters"=w451:string[][])  [unwired: 1 in]
        n91 = Delete From Array(array=w451, index (col)=0 ("disabled index (col)")) -> (array with subset deleted=w449:string[][])  [unwired: 2 in, 1 out]
        n92 = Bundle By Name(cluster=w448, "Statistical parameters"=w449, "RackID"=u8 0 ("DataLogger.StatisticalInfo.RackID")) -> (w441:T2)
        n93 = Unbundle By Name(w448) -> ("SystemParameters.SoftwareFeatures.DataLoggingEnable"=w442:bool, "SystemParameters.SoftwareFeatures.PopupOptions.CpCpkOnReelFinish"=w447:bool)
        n94 = case shown="True" w447 {
          tunnel: w441 -> [w469 w472]
          tunnel: [w470 w476] -> w446
          tunnel: w439 -> [w470 w474]
          tunnel: w440 -> [w468 w473]
          tunnel: [w469 w472] -> w445
          tunnel: [w468 w471] -> w444
          frame False {
          }
          frame True {
            n95 = call "Output_SM.vi"("SM Private Data in"=w473, "Output Cluster"=w472, "Receiver Name"="UI", "State"="UI: StatisticalParameters", "error in (no error)"=w474) -> ("SM Private Data out"=w471:refnum<class "Inspection Statemachine.lvclass">, "error out"=w476:errorcluster)  [unwired: 9 in]
          }
        }
        n96 = case shown="False" w442 {
          tunnel: w446 -> [w455 w460]
          tunnel: w445 -> [_ w458]
          tunnel: w444 -> [_ w459]
          tunnel: [w455 w463] -> w443
          frame False {
            # "DL Disable"
          }
          frame True {
            # "DL Enable"
            n97 = call "Output_SM.vi"("SM Private Data in"=w459, "Output Cluster"=w458, "Receiver Name"="DL", "State"="DL: StatisticalDetails", "error in (no error)"=w460) -> ("SM Private Data out"=w457:refnum<class "Inspection Statemachine.lvclass">, "error out"=w456:errorcluster)  [unwired: 9 in]
            n98 = Bundle By Name(cluster=w458, "StateMsgToDL"="Post") -> (w466:T2)
            n99 = call "Output_SM.vi"("SM Private Data in"=w457, "Output Cluster"=w466, "Receiver Name"="DL", "State"="DL: StateMessage", "error in (no error)"=w456) -> ("error out"=w463:errorcluster)  [unwired: 9 in, 1 out]
          }
        }
      }
      event User Event {
        n100 = event-data() -> ("ReelCount"=w481:u64, "TotalCount"=w480:u64)  [unwired: 1 in]
        n101 = Unbundle By Name(w484) -> ("OutputCluster"=w483:T2)
        n102 = Bundle By Name(cluster=w483, "IgnoredCountDetails.ReelCount"=w481, "IgnoredCountDetails.TotalCount"=w480) -> (w482:T2)
        n103 = call "Output_SM.vi"("SM Private Data in"=w485, "Output Cluster"=w482, "Receiver Name"="RC", "State"="RC: IgnoredCountDetails", "error in (no error)"=w488) -> ("error out"=w487:errorcluster)  [unwired: 9 in, 1 out]
      }
    }
  }
  "NextState" <- w18
  "LocalData_SM out" <- w5
  n104 = Unregister For Events(event registration refnum=w17, error in=w16) -> (error out=→"error out":errorcluster)
